vi "myRIO v1.0 Shutdown Writing DMA.vi"(8 "error in (no error)":errorcluster) -> (0 "error out":errorcluster)   [LabVIEW 2021]
uses:
  <vilib>/myRIO/Common/Instrument Driver Framework/Utilities/typedefs/Ref Counter Action Enum.ctl
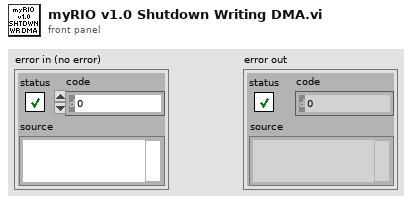
[diagram p1: front panel]
types:
  T1 = typedef "Ref Counter Action Enum.ctl" = enum16{"Set", "Get", "Increment", "Decrement"}
  T2 = typedef "Block Write Resource.ctl" = refnum<vi>
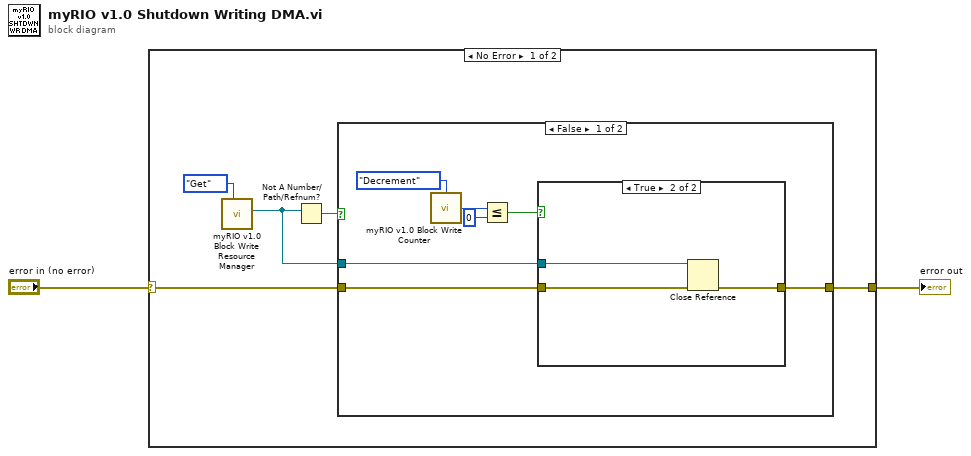
[diagram p0: block diagram]
diagram:
  n1 = case shown="No Error" "error in (no error)" {
    selector: "error in (no error)" -> [w5 w20]
    tunnel: [w4 w20] -> w1
    frame No Error {
      n2 = call <vilib>:"myRIO v1.0 Block Write Resource Manager.vi"("Action"=enum16{"Get", "Set", "Reset"}."Get") -> ("Resource Data Out"=w3:T2)  [unwired: 10 in]
      n3 = Not A Number/Path/Refnum?(number/path/refnum=w3) -> (NaN/Path/Refnum?=w6:bool)
      n4 = case shown="False" w6 {
        tunnel: w3 -> [w10 _]
        tunnel: w5 -> [w9 w19]
        tunnel: [w8 w19] -> w4
        frame False {
          n5 = call <vilib>:"myRIO v1.0 Block Write Counter.vi"("Resource Counter Action Enum"=Ref_Counter_Action_Enum."Decrement") -> ("Resource Count out"=w13:u32)  [unwired: 1 in]
          n6 = Less Or Equal?(x=w13, y=u32 0) -> (x <= y?=w11:bool)
          n7 = case shown="True" w11 {
            tunnel: w10 -> [_ w17]
            tunnel: w9 -> [w15 w16]
            tunnel: [w15 w18] -> w8
            frame False {
            }
            frame True {
              n8 = Close Reference(reference=w17, error in (no error)=w16) -> (error out=w18:errorcluster)
            }
          }
        }
        frame True {
        }
      }
    }
    frame Error {
    }
  }
  "error out" <- w1
